vi "test4.1-SyncMessage_Queue.vi"(8 "error in (no error)":errorcluster, 11 "TestCase in":refnum<class "testcase-CSMGlobalLog.lvclass">) -> (0 "error out":errorcluster, 3 "TestCase out":refnum<class "testcase-CSMGlobalLog.lvclass">)   [LabVIEW 2017, in "testcase-CSMGlobalLog.lvclass"]
uses:
  testcase-CSMGlobalLog.lvclass
  testcase-CSMGlobalLog.lvclass/testcase-CSMGlobalLog.ctl
  c9cb4a92-c6b2-48ff-9945-b938079fd949.vi
  <vilib>/addons/_JKI Toolkits/VI Tester/TestCase.llb/TestCase.lvclass
  src/user.lib/_NEVSTOP/Communicable State Machine(CSM)/Communicable State Machine.lvlib
  src/user.lib/_NEVSTOP/Communicable State Machine(CSM)/Utility/Periodic String Filter Setting.ctl
  C:/Program Files (x86)/National Instruments/LabVIEW 2017/vi.lib/addons/_JKI Toolkits/VI Tester/TestCase.llb/TestCase.lvclass
panel:
  out "String cache total":string
  out "size(s)":i32
  out "error out 2":errorcluster
  out "LoopCount":i32
  out "String Cache each loop":string
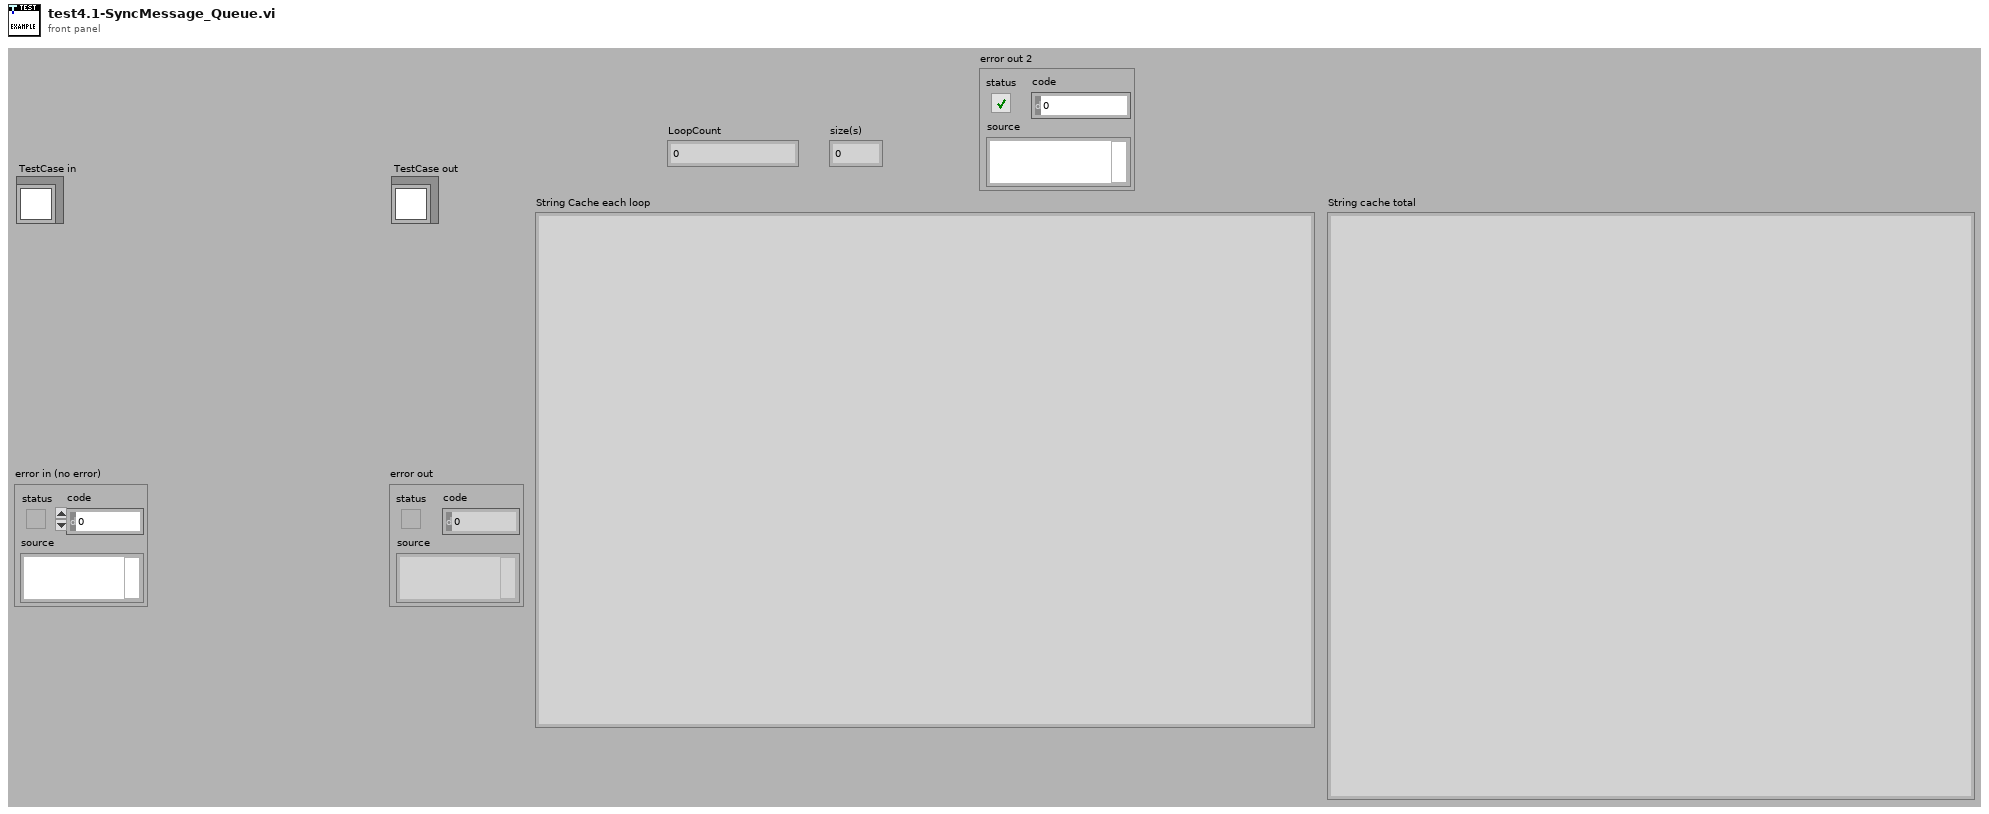
[diagram p1: front panel]
types:
  T1 = typedef "Communicable State Machine.lvlib/Periodic String Filter Setting.ctl" = cluster{"threashold(#/s)":dbl, "Check Peroid(s)":dbl}
  T2 = typedef "Communicable State Machine.lvlib/_CSM_GlobalLog_MSG.ctl" = cluster{"Name (\"\" to Use UUID)":string, "Current State":string, "Arguments":string, "Source Message":T3, "Source Module":string, "Complete(T)/Start(F)":bool, "LogType":T4, "Time Stamp":timestamp}
  T3 = typedef "Communicable State Machine.lvlib/_CSM_Response Source Message.ctl" = cluster{"‘State":string, "’Arguments":string, "’Error":errorcluster}
  T4 = typedef "Communicable State Machine.lvlib/_CSM_GlobalLog_MSG_TYPE.ctl" = enum16{"User Log", "State Change", "Status", "Interrupt", "Register", "Unregister", "Error Log", "Module Created", "Module Destroyed", "Async Message", "No-Rep Async Message", "Sync Message"}
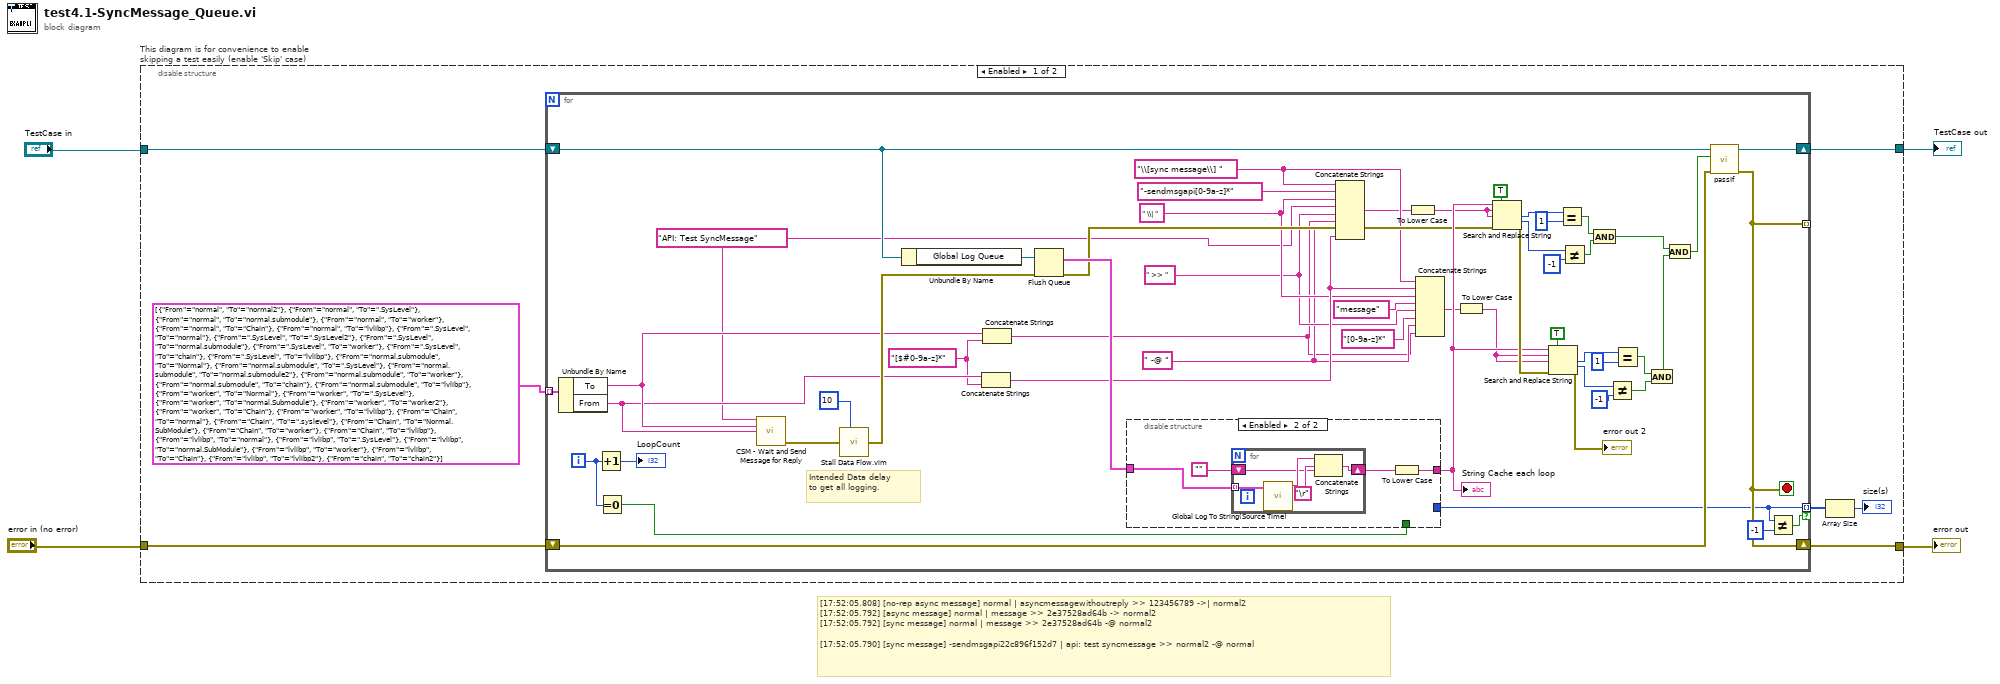
[diagram p0: block diagram]
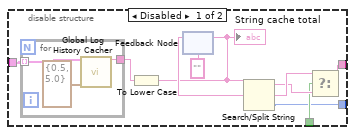
[diagram p2: hidden frame]
diagram:
  # "[17:52:05.808] [no-rep async message] normal | asyncmessagewithoutreply >> 123456789 ->| normal2\n[17:52:05.792] [async message] normal | message >> 2e37528ad64b -> normal2\n[17:52:05.792] [sync message] normal | message >> 2e37528ad64b -@ normal2\n\n[17:52:05.790] [sync message] -sendmsgapi22c896f152d7 | api: test syncmessage >> normal2 -@ normal"
  n1 = disable-structure "This diagram is for convenience to enable skipping a test easily (enable 'Skip' case)" shown="Enabled" {
    disable-tunnel: "TestCase in" -> [w8 w91]
    disable-tunnel: [w10 w89] -> w1
    disable-tunnel: [w11 w90] -> w3
    disable-tunnel: "error in (no error)" -> [w9 w88]
    frame Enabled {
      n2 = for {
        tunnel: cluster{"From":string, "To":string}[] [{"From"="normal", "To"="normal2"}, {"From"="normal", "To"=".SysLevel"}, {"From"="normal", "To"="normal.submodule"}, {"From"="normal", "To"="worker"}, {"From"="normal", "To"="Chain"}, {"From"="normal", "To"="lvlibp"}, {"From"=".SysLevel", "To"="normal"}, {"From"=".SysLevel", "To"=".SysLevel2"}, {"From"=".SysLevel", "To"="normal.submodule"}, {"From"=".SysLevel", "To"="worker"}, {"From"=".SysLevel", "To"="chain"}, {"From"=".SysLevel", "To"="lvlibp"}, {"From"="normal.submodule", "To"="Normal"}, {"From"="normal.submodule", "To"=".SysLevel"}, {"From"="normal.submodule", "To"="normal.submodule2"}, {"From"="normal.submodule", "To"="worker"}, {"From"="normal.submodule", "To"="chain"}, {"From"="normal.submodule", "To"="lvlibp"}, {"From"="worker", "To"="Normal"}, {"From"="worker", "To"=".SysLevel"}, {"From"="worker", "To"="normal.Submodule"}, {"From"="worker", "To"="worker2"}, {"From"="worker", "To"="Chain"}, {"From"="worker", "To"="lvlibp"}, {"From"="Chain", "To"="normal"}, {"From"="Chain", "To"=".syslevel"}, {"From"="Chain", "To"="Normal.SubModule"}, {"From"="Chain", "To"="worker"}, {"From"="Chain", "To"="lvlibp"}, {"From"="lvlibp", "To"="normal"}, {"From"="lvlibp", "To"=".SysLevel"}, {"From"="lvlibp", "To"="normal.SubModule"}, {"From"="lvlibp", "To"="worker"}, {"From"="lvlibp", "To"="Chain"}, {"From"="lvlibp", "To"="lvlibp2"}, {"From"="chain", "To"="chain2"}] -> [w43] mode=indexing
        shift-right: [w41] -> w11
        shift-left: w9 -> [w63]
        shift-right: [w65] -> w10
        shift-left: w8 -> [w42]
        tunnel: [w41] -> _ mode=indexing
        tunnel: [w30] -> w7 mode=indexing if=w40
        i -> [w38]
        stop <- w41 stop-if-true
        w12 = "[$#0-9a-z]*" ("string")
        w19 = " -@ "
        w21 = " >> "
        w23 = " \\| "
        w13 = "API: Test SyncMessage" ("State")
        w25 = "\\[sync message\\] "
        # "Intended Data delay\nto get all logging."
        n3 = Unbundle By Name(w43) -> ("To"=w27:string, "From"=w26:string)
        n4 = Increment(x=w38) -> (x+1=→"LoopCount":i32)
        n5 = Equal To 0?(x=w38) -> (x = 0?=w31:bool)
        n6 = call "CSM - Wait and Send Message for Reply.vi"("State"=w13, "Arguments (\"\")"=w27, "Target Module"=w26) -> ("error out"=w37:errorcluster)  [unwired: 9 in, 3 out]
        n7 = call "Stall Data Flow.vim"("value in"=w37, "milliseconds to wait"=u32 10 ("millisecond timer value")) -> ("value out"=w36:errorcluster)  [unwired: 1 out]
        n8 = Unbundle By Name(w42) -> ("Global Log Queue"=w64:refnum<queue>)
        n9 = Concatenate Strings(w26, w12) -> (w24:string)
        n10 = Concatenate Strings(w27, w12) -> (w18:string)
        n11 = Flush Queue(queue=w64, error in (no error)=w36) -> (remaining elements=w33:T2[], error out=w29:errorcluster)  [unwired: 1 out]
        n12 = disable-structure shown="Enabled" {
          disable-tunnel: [w69 w79] -> w32
          disable-tunnel: w31 -> [w68 _]
          disable-tunnel: w33 -> [w67 w81]
          disable-tunnel: [w66 _] -> w30
          frame Disabled {
            n13 = for {
              tunnel: w67 -> [w78] mode=indexing
              tunnel: [w77] -> w75
              n14 = call "Global Log History Cacher.vi"("Global Log Data"=w78, "Settings"=T1 {"threashold(#/s)"=0.5, "Check Peroid(s)"=5.0}) -> ("String Cache"=w77:string)  [unwired: 13 in]
            }
            n15 = To Lower Case(string=w75) -> (all lower case string=w70:string)
            "String cache total" <- w70
            n16 = feedback #1("") -> (w74:string)
            n17 = feedback-in #1(w70) -> ()
            n18 = Search/Split String(string=w70, search string/char (-)=w74) -> (substring before match=w71:string, match + rest of string=w72:string, offset of match=w66:i32)  [unwired: 1 in]
            n19 = Select(t=w72, s=w68, f=w71) -> (s? t:f=w69:string)
          }
          frame Enabled {
            n20 = for {
              tunnel: w81 -> [w87] mode=indexing
              shift-right: [w83] -> w80
              shift-left: "" -> [w84]
              n21 = call "Global Log To String(Source Time).vi"("Log"=w87) -> ("Log String"=w86:string)  [unwired: 9 in]
              n22 = Concatenate Strings(w86, "\r", w84) -> (w83:string)
            }
            n23 = To Lower Case(string=w80) -> (all lower case string=w79:string)
          }
        }
        "String Cache each loop" <- w32
        n24 = Concatenate Strings(w25, "-sendmsgapi[0-9a-z]*", w23, w13, w21, w18, w19, w24) -> (w17:string)
        n25 = To Lower Case(string=w17) -> (all lower case string=w16:string)
        n26 = Concatenate Strings(w25, w24, w23, "message", w21, "[0-9a-z]*", w19, w18) -> (w15:string)
        n27 = To Lower Case(string=w15) -> (all lower case string=w14:string)
        n28 = Search and Replace String(replace all?=TRUE ("replace all? (F)"), input string=w32, search string=w16, replace string=w16, error in=w29) -> (number of replacements=w60:i32, offset past replacement=w59:i32, error out=w49:errorcluster)  [unwired: 3 in, 1 out]
        n29 = Search and Replace String(replace all?=TRUE ("replace all? (F)"), input string=w32, search string=w14, replace string=w14, error in=w49) -> (number of replacements=w51:i32, offset past replacement=w52:i32, error out=→"error out 2":errorcluster)  [unwired: 3 in, 1 out]
        n30 = Equal?(x=w60, y=1) -> (x = y?=w57:bool)
        n31 = Not Equal?(x=w59, y=-1) -> (x != y?=w56:bool)
        n32 = And(x=w57, y=w56) -> (x .and. y?=w44:bool)
        n33 = Not Equal?(x=w52, y=-1) -> (x != y?=w55:bool)
        n34 = Equal?(x=w51, y=1) -> (x = y?=w54:bool)
        n35 = And(x=w54, y=w55) -> (x .and. y?=w48:bool)
        n36 = And(x=w44, y=w48) -> (x .and. y?=w34:bool)
        n37 = call-dynamic "passIf.vi"("error in (no error)"=w63, "pass"=w34, "TestCase in"=w42) -> ("error out"=w41:errorcluster, "TestCase out"=w65:refnum<class "testcase-CSMGlobalLog.lvclass">)  [unwired: 7 in]
        n38 = Not Equal?(x=w30, y=-1) -> (x != y?=w40:bool)
      }
      n39 = Array Size(array=w7) -> (size(s)=→"size(s)":i32)
    }
    frame Disabled {
      # "skip test result while test is under development"
      n40 = call <vilib>:"skip.vi"("error in (no error)"=w88, "TestCase in"=w91) -> ("error out"=w90:errorcluster, "TestCase out"=w89:refnum<class "testcase-CSMGlobalLog.lvclass">)  [unwired: 8 in]
    }
  }
  "error out" <- w3
  "TestCase out" <- w1
